vi "cubic predictor.vi"(9 "Limit Weight":dbl, 10 "Weights":dbl[](array[numeric])=[150.435262], 11 "Time":dbl[](array[numeric])=[14234.07814]) -> (2 "Best Polynomial Fit":dbl[](array[numeric]), 3 "Seconds to Completion":i32)   [LabVIEW 2009]
uses:
  <vilib>/Analysis/6fits.llb/Curve Fitting Criteria.ctl
  <vilib>/Analysis/NI_AALPro.lvlib
panel:
  out "Polynomial Coefficients":dbl[](array[numeric])
  out "Estimated Value":dbl
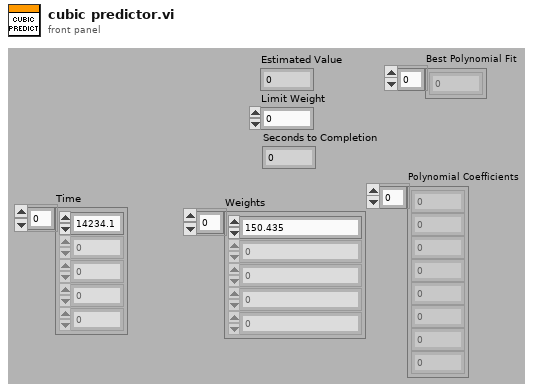
[diagram p1: front panel]
types:
  T1 = typedef "NI_AALPro.lvlib/Curve Fitting Criteria.ctl" = u16
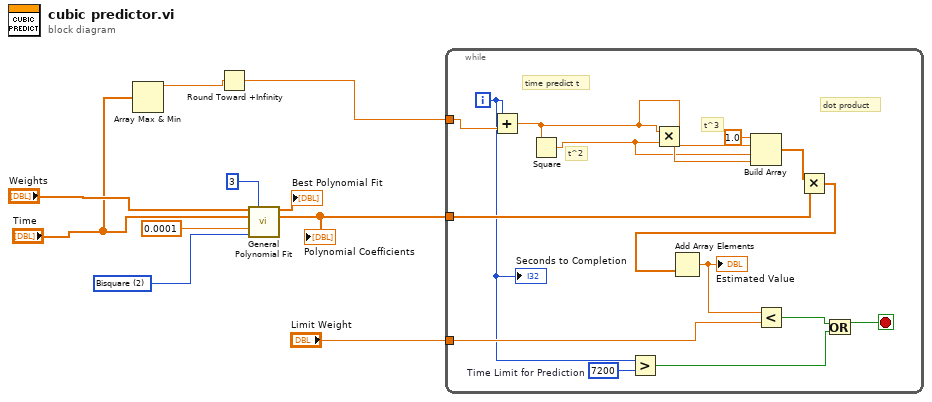
[diagram p0: block diagram]
diagram:
  w9 = T1 2 items=["Least Square", "Least Absolute Residual", "Bisquare"] ("method")
  n1 = Array Max & Min(array="Time") -> (max value=w7:dbl)  [unwired: 3 out]
  n2 = Round Toward +Infinity(x=w7) -> (ceil(x): smallest int >= x=w6:dbl)
  n3 = call <vilib>:"General Polynomial Fit.vi"("Y"="Weights", "polynomial order"=3, "X"="Time", "tolerance"=0.0001, "method"=w9) -> ("Best Polynomial Fit"=→"Best Polynomial Fit":dbl[], "Polynomial Coefficients"=w5:dbl[])  [unwired: 7 in, 2 out]
  "Polynomial Coefficients" <- w5
  n4 = while {
    tunnel: w6 -> [w25]
    tunnel: w5 -> [w19]
    tunnel: "Limit Weight" -> [w16]
    i -> [w14]
    stop <- w11 stop-if-true
    w13 = 7200  # Time Limit for Prediction
    # "dot product"
    # "t^3"
    # "t^2"
    # "time predict t"
    n5 = Add(x=w14, y=w25) -> (x+y=w21:dbl)
    n6 = Square(x=w21) -> (x^2=w22:dbl)
    n7 = Greater?(x=w14, y=w13) -> (0:w12:bool)
    n8 = Multiply(x=w21, y=w22) -> (x*y=w23:dbl)
    n9 = Build Array(1.0 ("element"), w21, w22, w23) -> (w20:dbl[])
    n10 = Multiply(x=w20, y=w19) -> (x*y=w18:dbl[])
    n11 = Add Array Elements(numeric array=w18) -> (sum=w17:dbl)
    "Estimated Value" <- w17
    n12 = Less?(x=w17, y=w16) -> (x < y?=w15:bool)
    n13 = Or(x=w15, y=w12) -> (x .or. y?=w11:bool)
    "Seconds to Completion" <- w14
  }
